vi "PJT_03.vi"() -> ()   [LabVIEW 2019]
uses:
  <vilib>/express/express shared/transition.llb/Dynamic To Waveform Array.vi
  <vilib>/express/express arith-compare/Formula/Block/exnFormulaBlock how many pts in the wave.vi
  <vilib>/express/express shared/ex_Modify Signal Name.vi
  <vilib>/express/express shared/transition.llb/Waveform Array To Dynamic.vi
  <vilib>/express/express arith-compare/Formula/XNode/ExpressFormulaBlockNode.xnode
panel:
  in  "정지":bool
  out "불리언 3":bool
  out "불리언 2":bool
  out "숫자형":dbl
  in  "불리언":bool
  out "웨이브폼 그래프 2":dynamicdata(graph)
  out "웨이브폼 그래프":dynamicdata(graph)
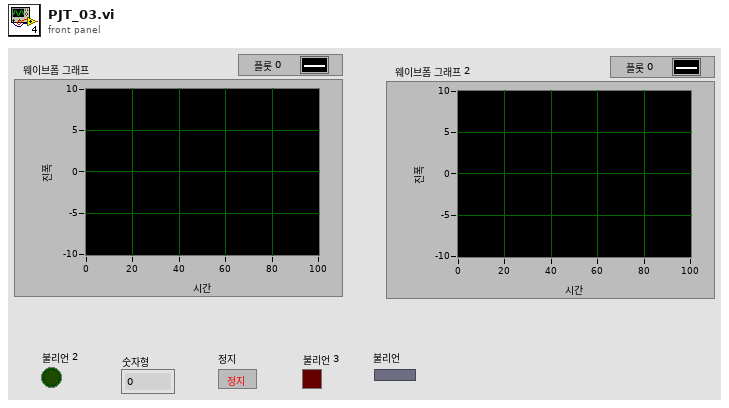
[diagram p1: front panel]
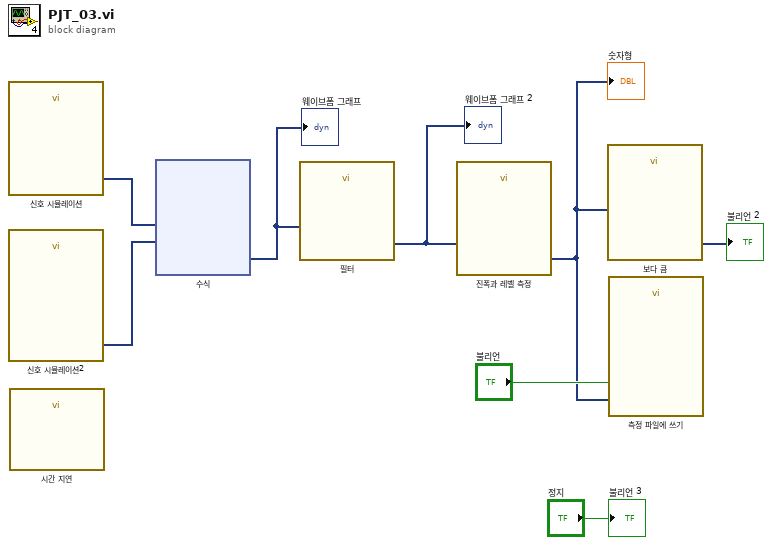
[diagram p0: block diagram]
diagram:
  n1 = call "신호 시뮬레이션"() -> ("사인파"=w8:dynamicdata)  [unwired: 14 in, 1 out]
  n2 = call "신호 시뮬레이션2"() -> ("60 Hz 및 노이즈"=w7:dynamicdata)  [unwired: 14 in, 1 out]
  n3 = call "시간 지연"() -> ()  [unwired: 11 in, 1 out]
  n4 = xnode "수식"("사인파"=w8, "60 Hz 및 노이즈"=w7) -> ("결과"=w6:dynamicdata)  [unwired: 1 in, 1 out]
  "웨이브폼 그래프" <- w6
  n5 = call "필터"("Signal"=w6) -> ("Filtered Signal"=w5:dynamicdata)  [unwired: 9 in, 1 out]
  "웨이브폼 그래프 2" <- w5
  n6 = call "진폭과 레벨 측정"("Signals"=w5) -> ("Peak to Peak"=w3:dynamicdata)  [unwired: 13 in, 1 out]
  "숫자형" <- w3
  n7 = call "보다 큼"("Operand 1"=w3) -> ("Result"=→"불리언 2":dynamicdata)  [unwired: 9 in, 1 out]
  n8 = call "측정 파일에 쓰기"("Signals"=w3, "Enable"="불리언") -> ()  [unwired: 15 in, 3 out]
  "불리언 3" <- "정지"
